vi "Set Font.vi"(8 "error in":errorcluster, 10 "Font.lvclass":refnum<class "Font.lvclass">, 11 "View in":refnum<class "Cell View.lvclass">) -> (0 "error out":errorcluster, 3 "View out":refnum<class "Cell View.lvclass">)   [LabVIEW 2023, in "SourceGrid.lvlib" / "Cell View.lvclass"]
uses:
  Cell View.lvclass
  Font/Font.lvclass
  Cell View.lvclass/Cell View.ctl
  D:/git/Sourcegrid-LabVIEW/dll/SourceGrid.dll
  dll/SourceGrid.dll
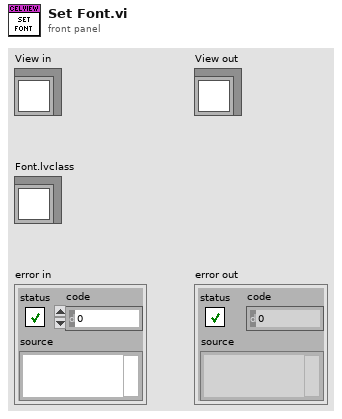
[diagram p1: front panel]
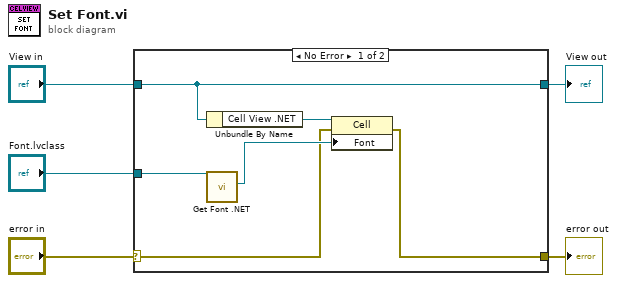
[diagram p0: block diagram]
diagram:
  n1 = case shown="No Error" "error in" {
    selector: "error in" -> [w8 w12]
    tunnel: [w7 w12] -> w4
    tunnel: [w6 w13] -> w2
    tunnel: "View in" -> [w6 w13]
    tunnel: "Font.lvclass" -> [w10 _]
    frame No Error {
      n2 = Unbundle By Name(w6) -> ("Cell View .NET"=w11:refnum<k24>)
      n3 = call "Get Font .NET.vi"("Font in"=w10) -> ("Font .NET"=w9:refnum<k24>)  [unwired: 9 in, 1 out]
      n4 = property class="Cell"(reference=w11, error in=w8, "Font"=w9) -> (error out=w7:errorcluster)  [unwired: 1 out]
    }
    frame Error {
    }
  }
  "error out" <- w4
  "View out" <- w2
